vi "Create Transfer Group Configuration.vi"(6 "group timing (dec:1, off: 0)":T3={"Decimation"=1, "Offset"=0}, 7 "base group name (group)":string="group", 9 "direction":T2, 10 "channel count per transfer":i32, 11 "transfers per group":i32) -> (3 "transfer group":T1={"name"="", "direction"=enum."Tx", "cycle timing"={"Decimation"=1, "Offset"=0}, "Transfers"=[]})   [LabVIEW 2017]
uses:
  Source/Shared/Typedefs/DSF.Shared.Typedefs.Cycle Timing Factors.ctl
  Source/Shared/Typedefs/DSF.Shared.Typedefs.Direction.ctl
  Source/Shared/Typedefs/DSF.Shared.Refactor.Typedefs.Transfer Group Configuration.Aggregate.ctl
  Source/Shared/Typedefs/DSF.Shared.Refactor.Typedefs.Transfer Configuration.ctl
  Source/Shared/Typedefs/DSF.Shared.Typedefs.Byte Order.ctl
  Source/Shared/Typedefs/DSF.Shared.Refactor.Typedefs.Channel Array Configuration.ctl
  Source/Shared/Typedefs/DSF.Shared.Typedefs.Data Type.ctl
  Source/DSF.Shared.lvlib
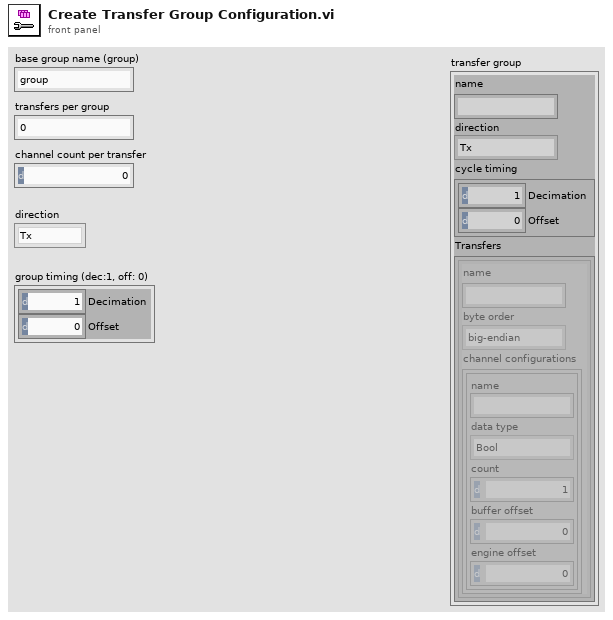
[diagram p1: front panel]
types:
  T1 = typedef "DSF.Shared.lvlib/DSF.Shared.Refactor.Typedefs.Transfer Group Configuration.Aggregate.ctl" = cluster{"name":string, "direction":T2, "cycle timing":T3, "Transfers":T4[]}
  T2 = typedef "DSF.Shared.lvlib/DSF.Shared.Typedefs.Direction.ctl" = enum8{"Tx", "Rx"}
  T3 = typedef "DSF.Shared.lvlib/DSF.Shared.Typedefs.Cycle Timing Factors.ctl" = cluster{"Decimation":u64, "Offset":u64}
  T4 = typedef "DSF.Shared.lvlib/DSF.Shared.Refactor.Typedefs.Transfer Configuration.ctl" = cluster{"name":string, "byte order":T5, "channel configurations":T6[]}
  T5 = typedef "DSF.Shared.lvlib/DSF.Shared.Typedefs.Byte Order.ctl" = enum8{"big-endian", "little-endian"}
  T6 = typedef "DSF.Shared.lvlib/DSF.Shared.Refactor.Typedefs.Channel Array Configuration.ctl" = cluster{"name":string, "data type":T7, "count":u64, "buffer offset":u64, "engine offset":u64}
  T7 = typedef "DSF.Shared.lvlib/DSF.Shared.Typedefs.Data Type.ctl" = enum8{"Bool", "SGL", "DBL", "I8", "I16", "I32", "I64", "U8", "U16", "U32", "U64"}
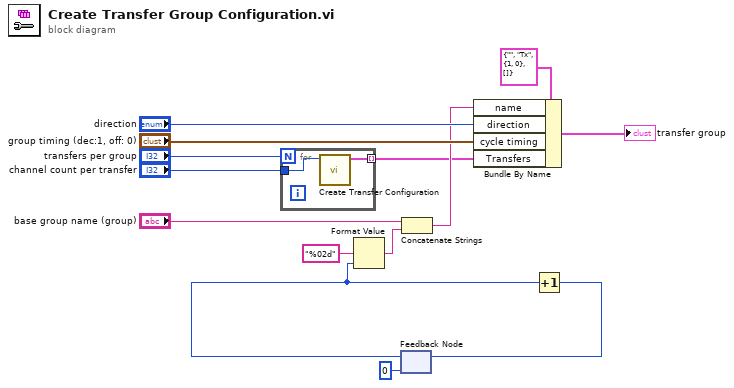
[diagram p0: block diagram]
diagram:
  n1 = for {
    N: "transfers per group" -> [_]
    tunnel: "channel count per transfer" -> [w16]
    tunnel: [w15] -> w1 mode=indexing
    n2 = call "Create Transfer Configuration.vi"("channel count per transfer"=w16) -> ("transfer configuration"=w15:T4)  [unwired: 10 in]
  }
  n3 = feedback #1(0) -> (w11:i32)
  n4 = Format Value(format string="%02d", value (0)=w11) -> (output string=w3:string)  [unwired: 1 in]
  n5 = Concatenate Strings("base group name (group)", w3) -> (w2:string)
  n6 = Bundle By Name(cluster=T1 {"name"="", "direction"=enum."Tx", "cycle timing"={"Decimation"=1, "Offset"=0}, "Transfers"=[]} ("Transfer Group Configuration"), "name"=w2, "direction"="direction", "cycle timing"="group timing (dec:1, off: 0)", "Transfers"=w1) -> (→"transfer group":T1)
  n7 = Increment(x=w11) -> (x+1=w9:i32)
  n8 = feedback-in #1(w9) -> ()
